vi "Write Sensor Parameters.vi"(4 "Sensor_false_positive":dbl, 6 "Sensor_true_negative":dbl, 8 "error in (no error)":errorcluster, 9 "Sensor_false_negative":dbl, 10 "Sensor_true_positive":dbl, 11 "Probabilistic_OccupancyGrid in":refnum<class "Probabilistic_OccupancyGrid.lvclass">) -> (0 "error out":errorcluster, 3 "Probabilistic_OccupancyGrid out":refnum<class "Probabilistic_OccupancyGrid.lvclass">)   [LabVIEW 2017, in "Probabilistic_OccupancyGrid.lvclass"]
uses:
  Probabilistic_OccupancyGrid.lvclass
  Probabilistic_OccupancyGrid.lvclass/Probabilistic_OccupancyGrid.ctl
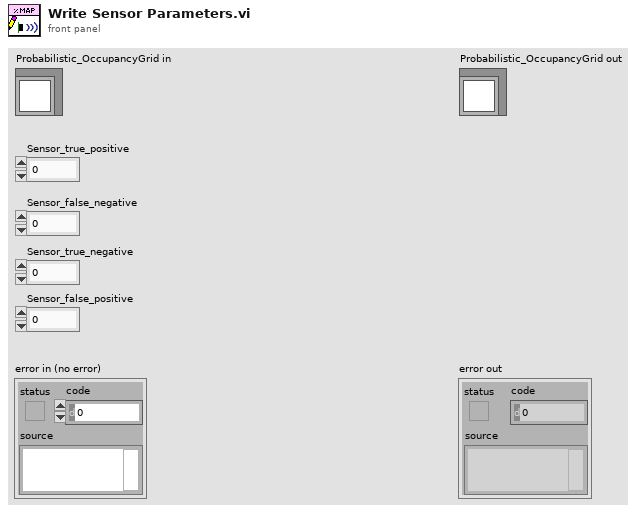
[diagram p1: front panel]
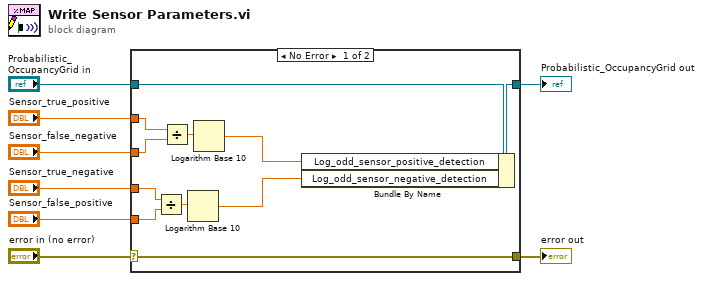
[diagram p0: block diagram]
diagram:
  n1 = case shown="No Error" "error in (no error)" {
    selector: "error in (no error)" -> [w19 w20]
    tunnel: [w19 w20] -> w7
    tunnel: [w17 w21] -> w5
    tunnel: "Probabilistic_OccupancyGrid in" -> [w18 w21]
    tunnel: "Sensor_true_positive" -> [w15 _]
    tunnel: "Sensor_false_negative" -> [w14 _]
    tunnel: "Sensor_true_negative" -> [w11 _]
    tunnel: "Sensor_false_positive" -> [w10 _]
    frame No Error {
      n2 = Divide(x=w11, y=w10) -> (x/y=w12:dbl)
      n3 = Divide(x=w15, y=w14) -> (x/y=w16:dbl)
      n4 = Logarithm Base 10(1:w12) -> (0:w9:dbl)
      n5 = Logarithm Base 10(1:w16) -> (0:w13:dbl)
      n6 = Bundle By Name(cluster=w18, "Log_odd_sensor_positive_detection"=w13, "Log_odd_sensor_negative_detection"=w9) -> (w17:refnum<class "Probabilistic_OccupancyGrid.lvclass">)
    }
    frame Error {
    }
  }
  "error out" <- w7
  "Probabilistic_OccupancyGrid out" <- w5
